vi "Pi-Plate Demo Min.vi"() -> ()   [LabVIEW 2025]
panel:
  out "Waveform Chart":dbl(graph)
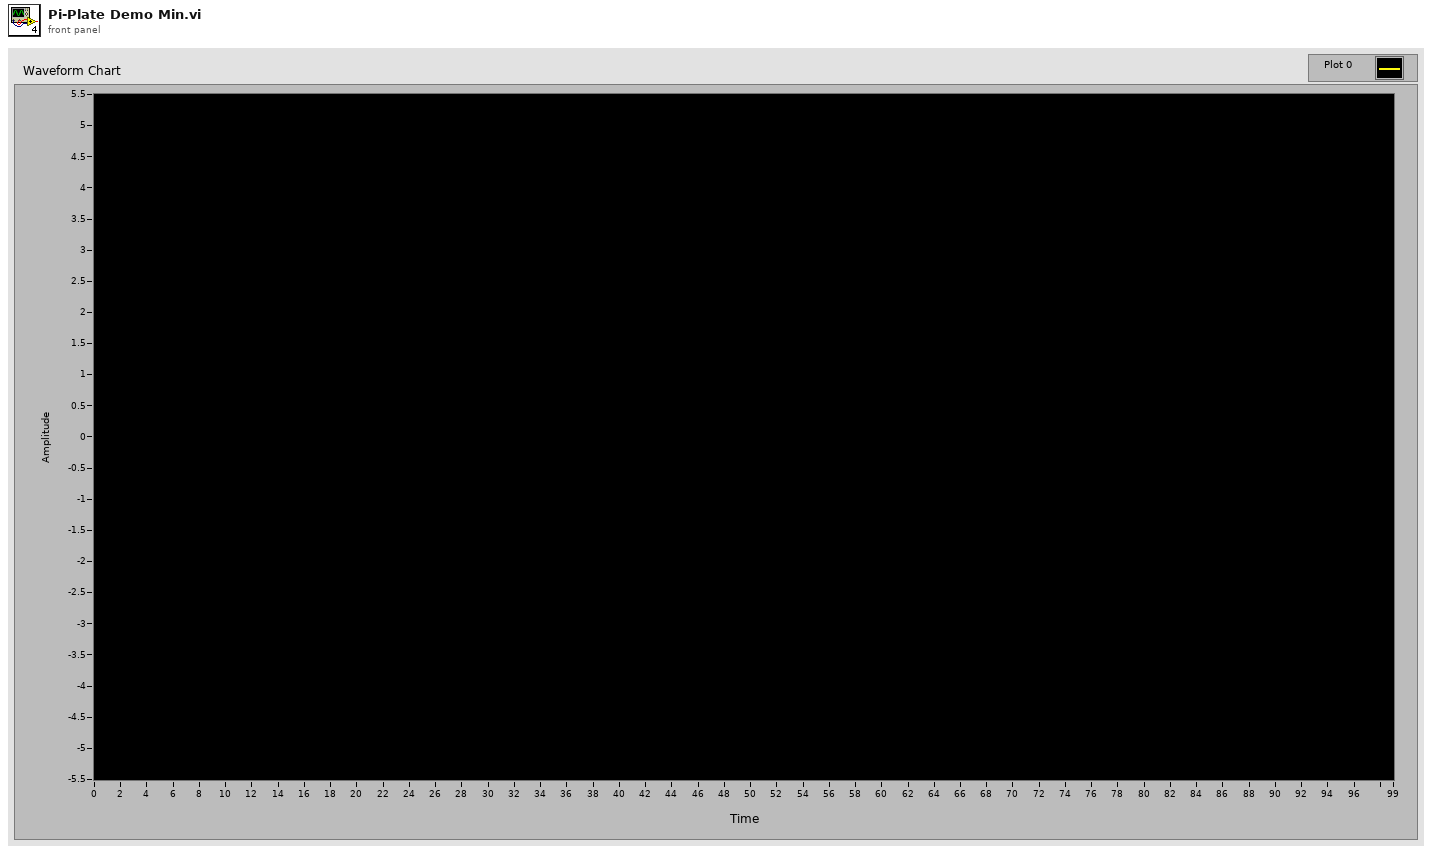
[diagram p1: front panel]
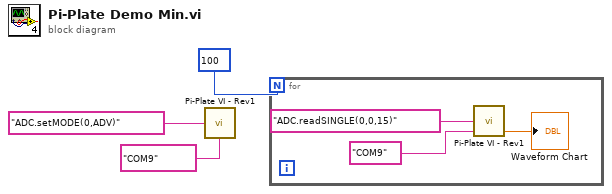
[diagram p0: block diagram]
diagram:
  n1 = call "Pi-Plate VI - Rev1.vi"("Pi-Plate Command"="ADC.setMODE(0,ADV)", "COM Port"="COM9") -> ()  [unwired: 3 in, 3 out]
  n2 = for {
    N: 100 -> [_]
    n3 = call "Pi-Plate VI - Rev1.vi"("Pi-Plate Command"="ADC.readSINGLE(0,0,15)", "COM Port"="COM9") -> ("Numeric Value"=→"Waveform Chart":dbl)  [unwired: 3 in, 2 out]
  }
